vi "round_at_dec (SubVI).vi"(8 "Decimal":dbl, 11 "numeric in":dbl) -> (3 "Numeric out":dbl)   [LabVIEW 2024]
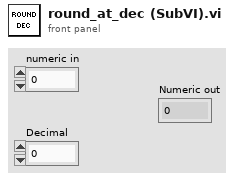
[diagram p1: front panel]
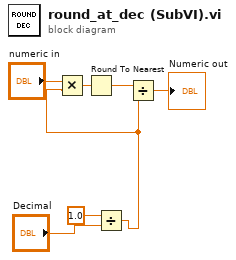
[diagram p0: block diagram]
diagram:
  n1 = Divide(x=1.0, y="Decimal") -> (x/y=w3:dbl)
  n2 = Multiply(x="numeric in", y=w3) -> (x*y=w2:dbl)
  n3 = Round To Nearest(number=w2) -> (nearest integer value=w6:dbl)
  n4 = Divide(x=w6, y=w3) -> (x/y=→"Numeric out":dbl)
